vi "Get Lamp Voltage.vi"(8 "error in (no error)":errorcluster, 11 "Neph in":refnum<class "Nephelometer.lvclass">) -> (0 "error out":errorcluster, 2 "Lamp Data":cluster{"Voltage":dbl, "Amperage":dbl}, 3 "Neph out":refnum<class "Nephelometer.lvclass">)   [LabVIEW 2014, in "Nephelometer.lvclass"]
uses:
  Nephelometer.lvclass
  Nephelometer.lvclass/Nephelometer.ctl
  Reusable/Session APIs/Serial/Public/Get Data/Get String.vi
  Reusable/Session APIs/Text Communication/Text Device Session.lvclass
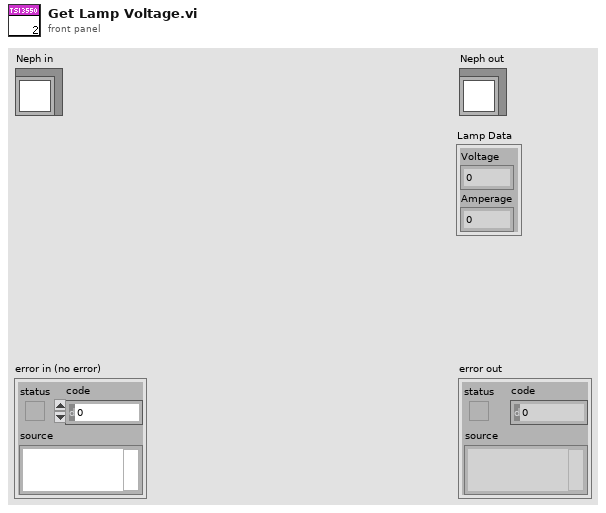
[diagram p1: front panel]
types:
  T1 = typedef "Session - Root.lvclass/Session Handle.ctl" = refnum<data-value>
  T2 = cluster{"array type (2D Dbl)[0]":dbl, "array type (2D Dbl)[1]":dbl}
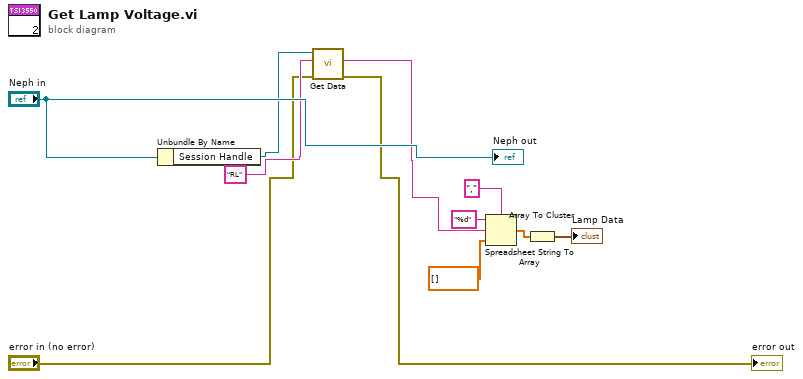
[diagram p0: block diagram]
diagram:
  n1 = Unbundle By Name("Neph in") -> ("Session Handle"=w4:T1)
  n2 = call-poly "Get Data.vi"("error in"="error in (no error)", "CMD"="RL", "handle in"=w4) -> ("error out"=→"error out":errorcluster, "DataOut"=w3:string)  [unwired: 6 in, 1 out]
  n3 = Spreadsheet String To Array(delimiter (Tab)=",", format string="%d", spreadsheet string=w3, array type (2D Dbl)=dbl[] []) -> (array=w7:dbl[])
  n4 = Array To Cluster(array=w7) -> (cluster=→"Lamp Data":T2)
  "Neph out" <- "Neph in"
